vi "4461 - AI Read Data.vi"(8 "error in (no error)":errorcluster, 9 "sampling info":cluster{"Fs":dbl, "#s":dbl}={"Fs"=1000.0, "#s"=1000.0} {"Fs" format="%.2p"}, 10 "AI Block Size":i32=5000, 11 "AI task":refnum<k21>[](array[refnum])=["", ""]) -> (0 "error out":errorcluster, 1 "Backlog":u8(slide) scale=0.0..100.0, 2 "Input Signals":dbl[][](array[numeric]), 3 "Input Signals":waveform(dbl)[](array[waveform]))   [LabVIEW 2013]
uses:
  <vilib>/DAQmx/read.llb/DAQmx Read (Analog 1D Wfm NChan NSamp).vi
  <vilib>/DAQmx/miscellaneous.llb/DAQmx Fill In Error Info.vi
  <resource>/objmgr/daqmx.rc
panel:
  out "AvailSampPerChan 8":u32
  out "AvailSampPerChan 7":u32
  out "AvailSampPerChan 6":u32
  out "AvailSampPerChan 5":u32
  out "AvailSampPerChan 4":u32
  out "AvailSampPerChan 3":u32
  out "AvailSampPerChan 2":u32
  out "AvailSampPerChan":u32
  in  "AI Rate":dbl=10000.0 format="%.2f"
  in  "AI Buffer Size (s)":i32=10
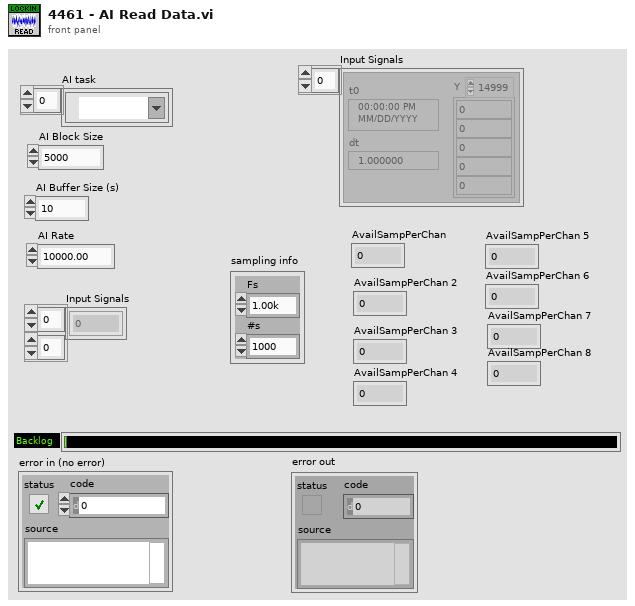
[diagram p1: front panel]
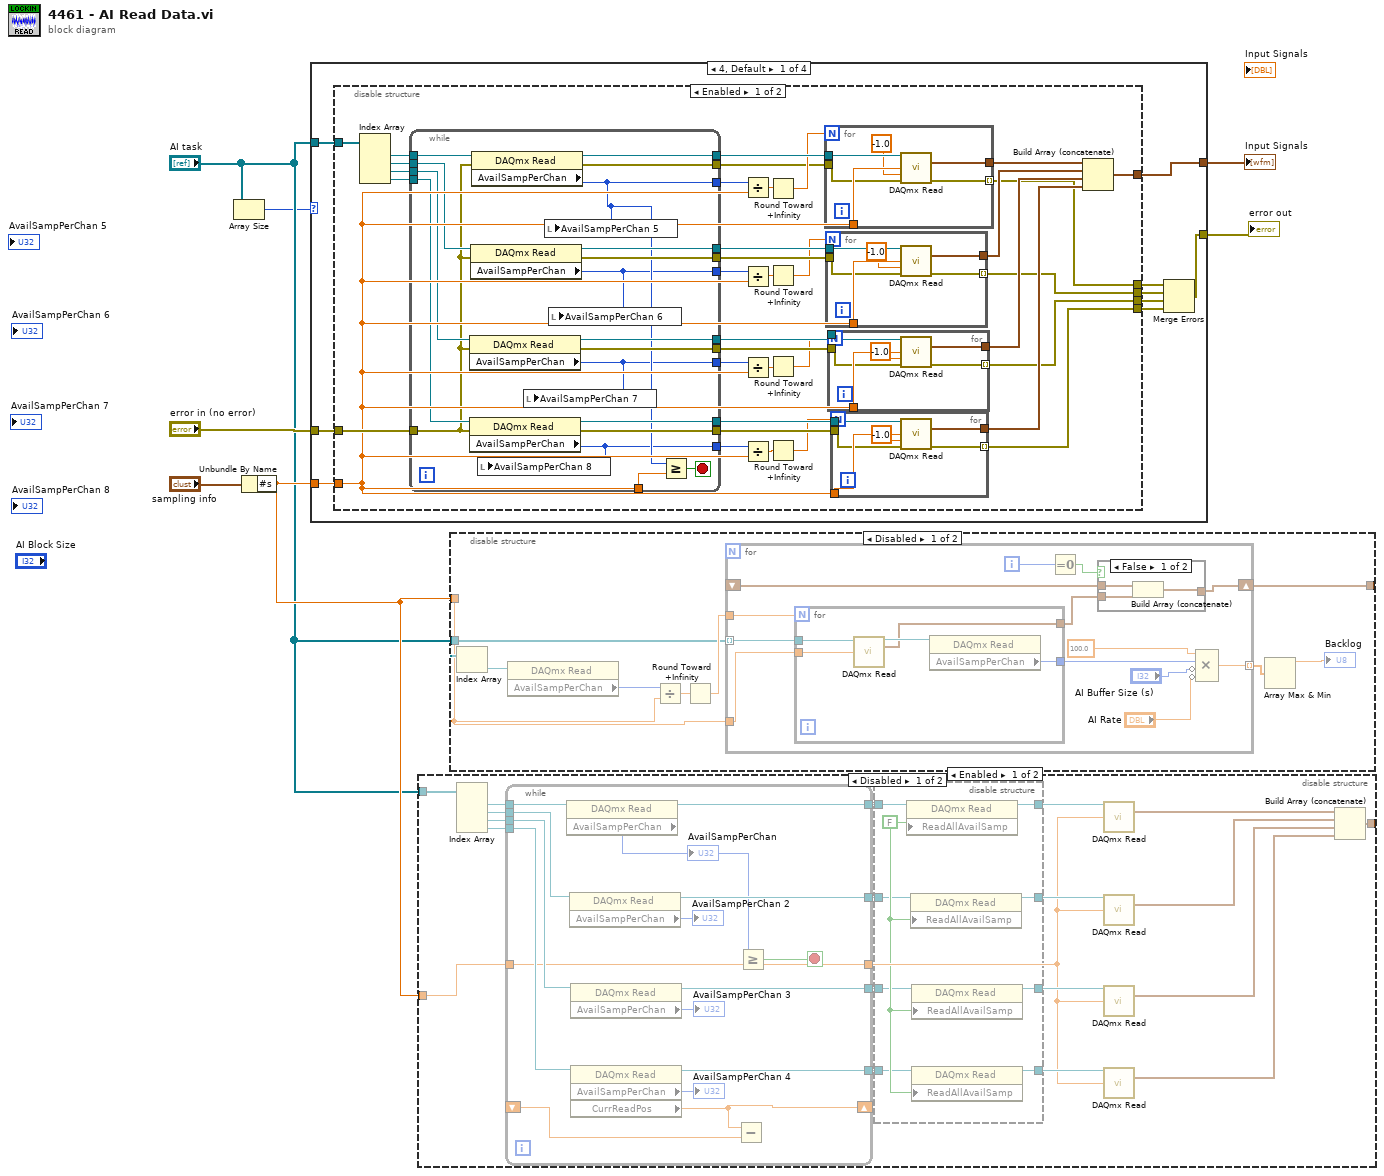
[diagram p0: block diagram]
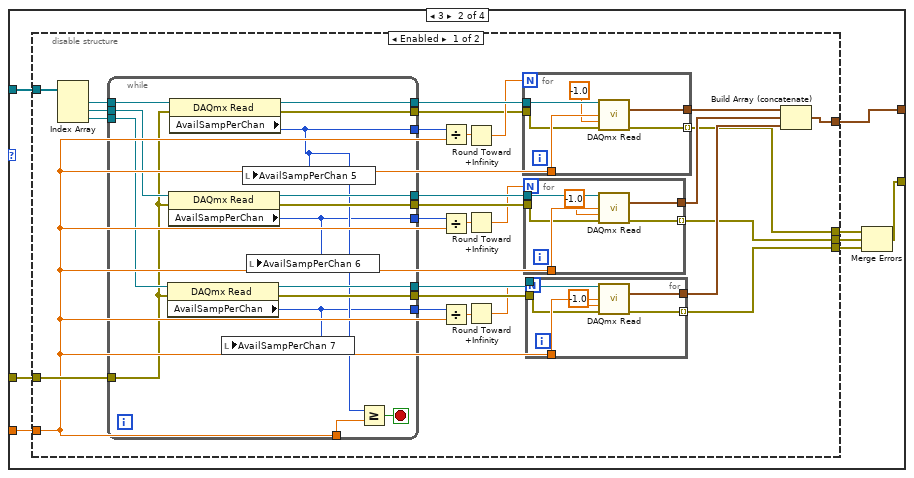
[diagram p3: hidden frame]
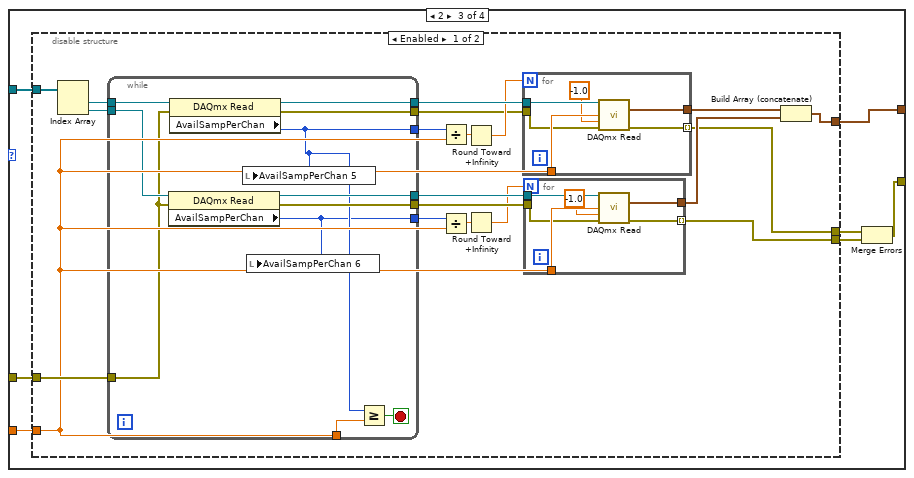
[diagram p5: hidden frame]
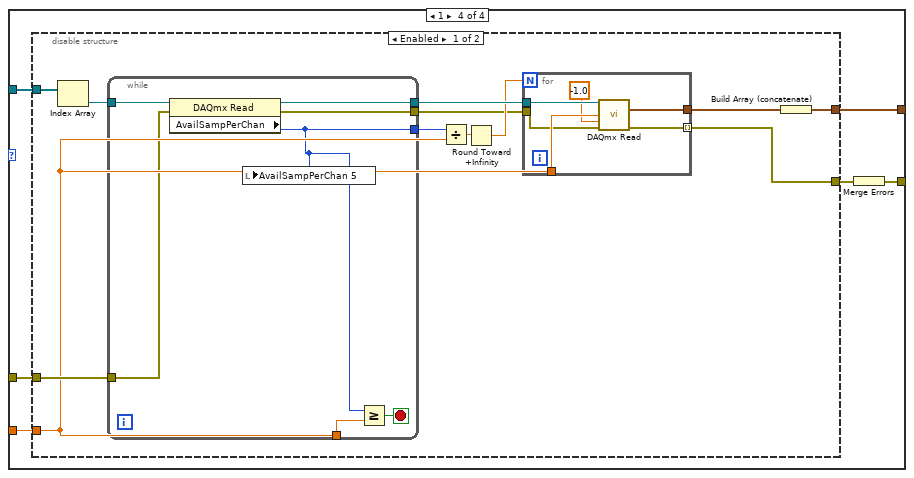
[diagram p7: hidden frame]
diagram:
  n1 = Array Size(array="AI task") -> (size(s)=w1:i32)
  n2 = Unbundle By Name("sampling info") -> ("#s"=w3:dbl)
  n3 = case shown="4, Default" w1 {
    tunnel: "AI task" -> [w16 w103 w171 w220]
    tunnel: [w15 w102 w170 w219] -> w6
    tunnel: "error in (no error)" -> [w14 w101 w169 w218]
    tunnel: [w12 w99 w167 w216] -> w4
    tunnel: w3 -> [w8 w96 w165 w215]
    frame 4, Default {
      n4 = disable-structure shown="Enabled" {
        disable-tunnel: w16 -> [w52 _]
        disable-tunnel: w8 -> [w17 _]
        disable-tunnel: [w31 _] -> w15
        disable-tunnel: w14 -> [w29 _]
        disable-tunnel: [w24 _] -> w13
        disable-tunnel: [w23 _] -> w11
        disable-tunnel: [w22 _] -> w10
        disable-tunnel: [w21 _] -> w9
        frame Enabled {
          n5 = Index Array(array=w52) -> (element #1=w44:refnum<k21>, element #2=w45:refnum<k21>, element #3=w46:refnum<k21>, element #4=w47:refnum<k21>)  [unwired: 4 in]
          n6 = while {
            tunnel: w47 -> [w71]
            tunnel: w46 -> [w70]
            tunnel: w45 -> [w69]
            tunnel: w44 -> [w68]
            tunnel: [w67] -> w43
            tunnel: [w66] -> w42
            tunnel: [w65] -> w41
            tunnel: [w64] -> w40
            tunnel: [w56] -> w39
            tunnel: [w53] -> w38
            tunnel: [w54] -> w37
            tunnel: [w55] -> w36
            tunnel: w29 -> [w57]
            tunnel: [w63] -> w28
            tunnel: [w62] -> w27
            tunnel: [w61] -> w26
            tunnel: [w60] -> w25
            tunnel: w17 -> [w59]
            stop <- w58 stop-if-true
            n7 = property class="DAQmx Read"(reference=w70, error in=w57) -> (reference out=w65:refnum<k21>, error out=w61:errorcluster, "AvailSampPerChan"=w54:u32)
            n8 = property class="DAQmx Read"(reference=w71, error in=w57) -> (reference out=w64:refnum<k21>, error out=w60:errorcluster, "AvailSampPerChan"=w53:u32)
            n9 = property class="DAQmx Read"(reference=w69, error in=w57) -> (reference out=w66:refnum<k21>, error out=w62:errorcluster, "AvailSampPerChan"=w55:u32)
            n10 = property class="DAQmx Read"(reference=w68, error in=w57) -> (reference out=w67:refnum<k21>, error out=w63:errorcluster, "AvailSampPerChan"=w56:u32)
            n11 = local write "AvailSampPerChan 8"(w53) -> ()
            n12 = local write "AvailSampPerChan 7"(w54) -> ()
            n13 = local write "AvailSampPerChan 5"(w56) -> ()
            n14 = local write "AvailSampPerChan 6"(w55) -> ()
            n15 = Greater Or Equal?(x=w56, y=w59) -> (x >= y?=w58:bool)
          }
          n16 = Divide(x=w39, y=w17) -> (x/y=w35:dbl)
          n17 = Divide(x=w36, y=w17) -> (x/y=w34:dbl)
          n18 = Divide(x=w37, y=w17) -> (x/y=w33:dbl)
          n19 = Divide(x=w38, y=w17) -> (x/y=w32:dbl)
          n20 = Round Toward +Infinity(x=w35) -> (ceil(x): smallest int >= x=w30:dbl)
          n21 = Round Toward +Infinity(x=w34) -> (ceil(x): smallest int >= x=w18:dbl)
          n22 = Round Toward +Infinity(x=w33) -> (ceil(x): smallest int >= x=w19:dbl)
          n23 = Round Toward +Infinity(x=w32) -> (ceil(x): smallest int >= x=w20:dbl)
          n24 = for {
            N: w30 -> [_]
            tunnel: [w95] -> w48
            tunnel: w43 -> [w94]
            tunnel: w17 -> [w93]
            tunnel: w28 -> [w92]
            tunnel: [w91] -> w24 mode=indexing
            n25 = call-poly <vilib>:"DAQmx Read.vi"("task/channels in"=w94, "number of samples per channel"=w93, "timeout"=-1.0, "error in"=w92) -> ("data"=w95:waveform(dbl)[], "error out"=w91:errorcluster)  [unwired: 9 in, 1 out]
          }
          n26 = for {
            N: w18 -> [_]
            tunnel: [w89] -> w49
            tunnel: w42 -> [w88]
            tunnel: w17 -> [w87]
            tunnel: w27 -> [w86]
            tunnel: [w85] -> w23 mode=indexing
            n27 = call-poly <vilib>:"DAQmx Read.vi"("task/channels in"=w88, "number of samples per channel"=w87, "timeout"=-1.0, "error in"=w86) -> ("data"=w89:waveform(dbl)[], "error out"=w85:errorcluster)  [unwired: 9 in, 1 out]
          }
          n28 = for {
            N: w19 -> [_]
            tunnel: [w83] -> w50
            tunnel: w41 -> [w82]
            tunnel: w17 -> [w81]
            tunnel: w26 -> [w80]
            tunnel: [w79] -> w22 mode=indexing
            n29 = call-poly <vilib>:"DAQmx Read.vi"("task/channels in"=w82, "number of samples per channel"=w81, "timeout"=-1.0, "error in"=w80) -> ("data"=w83:waveform(dbl)[], "error out"=w79:errorcluster)  [unwired: 9 in, 1 out]
          }
          n30 = for {
            N: w20 -> [_]
            tunnel: [w77] -> w51
            tunnel: w40 -> [w76]
            tunnel: w17 -> [w75]
            tunnel: w25 -> [w74]
            tunnel: [w73] -> w21 mode=indexing
            n31 = call-poly <vilib>:"DAQmx Read.vi"("task/channels in"=w76, "number of samples per channel"=w75, "timeout"=-1.0, "error in"=w74) -> ("data"=w77:waveform(dbl)[], "error out"=w73:errorcluster)  [unwired: 9 in, 1 out]
          }
          n32 = Build Array (concatenate)(w48, w49, w50, w51) -> (w31:waveform(dbl)[])
        }
        frame Disabled {
        }
      }
      n33 = Merge Errors(w13, w11, w10, w9) -> (w12:errorcluster)
    }
    frame 3 {
      n34 = disable-structure shown="Enabled" {
        disable-tunnel: w103 -> [w131 _]
        disable-tunnel: w96 -> [w104 _]
        disable-tunnel: [w115 _] -> w102
        disable-tunnel: w101 -> [w113 _]
        disable-tunnel: [w109 _] -> w100
        disable-tunnel: [w108 _] -> w98
        disable-tunnel: [w107 _] -> w97
        frame Enabled {
          n35 = Index Array(array=w131) -> (element #1=w125:refnum<k21>, element #2=w126:refnum<k21>, element #3=w127:refnum<k21>)  [unwired: 3 in]
          n36 = while {
            tunnel: w127 -> [w146]
            tunnel: w126 -> [w145]
            tunnel: w125 -> [w144]
            tunnel: [w143] -> w124
            tunnel: [w142] -> w123
            tunnel: [w141] -> w122
            tunnel: [w134] -> w121
            tunnel: [w132] -> w120
            tunnel: [w133] -> w119
            tunnel: w113 -> [w135]
            tunnel: [w140] -> w112
            tunnel: [w139] -> w111
            tunnel: [w138] -> w110
            tunnel: w104 -> [w137]
            stop <- w136 stop-if-true
            n37 = property class="DAQmx Read"(reference=w146, error in=w135) -> (reference out=w141:refnum<k21>, error out=w138:errorcluster, "AvailSampPerChan"=w132:u32)
            n38 = property class="DAQmx Read"(reference=w145, error in=w135) -> (reference out=w142:refnum<k21>, error out=w139:errorcluster, "AvailSampPerChan"=w133:u32)
            n39 = property class="DAQmx Read"(reference=w144, error in=w135) -> (reference out=w143:refnum<k21>, error out=w140:errorcluster, "AvailSampPerChan"=w134:u32)
            n40 = local write "AvailSampPerChan 7"(w132) -> ()
            n41 = local write "AvailSampPerChan 5"(w134) -> ()
            n42 = local write "AvailSampPerChan 6"(w133) -> ()
            n43 = Greater Or Equal?(x=w134, y=w137) -> (x >= y?=w136:bool)
          }
          n44 = Divide(x=w121, y=w104) -> (x/y=w118:dbl)
          n45 = Divide(x=w119, y=w104) -> (x/y=w117:dbl)
          n46 = Divide(x=w120, y=w104) -> (x/y=w116:dbl)
          n47 = Round Toward +Infinity(x=w118) -> (ceil(x): smallest int >= x=w114:dbl)
          n48 = Round Toward +Infinity(x=w117) -> (ceil(x): smallest int >= x=w105:dbl)
          n49 = Round Toward +Infinity(x=w116) -> (ceil(x): smallest int >= x=w106:dbl)
          n50 = for {
            N: w114 -> [_]
            tunnel: [w164] -> w128
            tunnel: w124 -> [w163]
            tunnel: w104 -> [w162]
            tunnel: w112 -> [w161]
            tunnel: [w160] -> w109 mode=indexing
            n51 = call-poly <vilib>:"DAQmx Read.vi"("task/channels in"=w163, "number of samples per channel"=w162, "timeout"=-1.0, "error in"=w161) -> ("data"=w164:waveform(dbl)[], "error out"=w160:errorcluster)  [unwired: 9 in, 1 out]
          }
          n52 = for {
            N: w105 -> [_]
            tunnel: [w158] -> w129
            tunnel: w123 -> [w157]
            tunnel: w104 -> [w156]
            tunnel: w111 -> [w155]
            tunnel: [w154] -> w108 mode=indexing
            n53 = call-poly <vilib>:"DAQmx Read.vi"("task/channels in"=w157, "number of samples per channel"=w156, "timeout"=-1.0, "error in"=w155) -> ("data"=w158:waveform(dbl)[], "error out"=w154:errorcluster)  [unwired: 9 in, 1 out]
          }
          n54 = for {
            N: w106 -> [_]
            tunnel: [w152] -> w130
            tunnel: w122 -> [w151]
            tunnel: w104 -> [w150]
            tunnel: w110 -> [w149]
            tunnel: [w148] -> w107 mode=indexing
            n55 = call-poly <vilib>:"DAQmx Read.vi"("task/channels in"=w151, "number of samples per channel"=w150, "timeout"=-1.0, "error in"=w149) -> ("data"=w152:waveform(dbl)[], "error out"=w148:errorcluster)  [unwired: 9 in, 1 out]
          }
          n56 = Build Array (concatenate)(w128, w129, w130) -> (w115:waveform(dbl)[])
        }
        frame Disabled {
        }
      }
      n57 = Merge Errors(w100, w98, w97) -> (w99:errorcluster)
    }
    frame 2 {
      n58 = disable-structure shown="Enabled" {
        disable-tunnel: w171 -> [w191 _]
        disable-tunnel: w165 -> [w172 _]
        disable-tunnel: [w180 _] -> w170
        disable-tunnel: w169 -> [w178 _]
        disable-tunnel: [w175 _] -> w168
        disable-tunnel: [w174 _] -> w166
        frame Enabled {
          n59 = Index Array(array=w191) -> (element #1=w187:refnum<k21>, element #2=w188:refnum<k21>)  [unwired: 2 in]
          n60 = while {
            tunnel: w188 -> [w202]
            tunnel: w187 -> [w201]
            tunnel: [w200] -> w186
            tunnel: [w199] -> w185
            tunnel: [w193] -> w184
            tunnel: [w192] -> w183
            tunnel: w178 -> [w194]
            tunnel: [w198] -> w177
            tunnel: [w197] -> w176
            tunnel: w172 -> [w196]
            stop <- w195 stop-if-true
            n61 = property class="DAQmx Read"(reference=w202, error in=w194) -> (reference out=w199:refnum<k21>, error out=w197:errorcluster, "AvailSampPerChan"=w192:u32)
            n62 = property class="DAQmx Read"(reference=w201, error in=w194) -> (reference out=w200:refnum<k21>, error out=w198:errorcluster, "AvailSampPerChan"=w193:u32)
            n63 = local write "AvailSampPerChan 5"(w193) -> ()
            n64 = local write "AvailSampPerChan 6"(w192) -> ()
            n65 = Greater Or Equal?(x=w193, y=w196) -> (x >= y?=w195:bool)
          }
          n66 = Divide(x=w184, y=w172) -> (x/y=w182:dbl)
          n67 = Divide(x=w183, y=w172) -> (x/y=w181:dbl)
          n68 = Round Toward +Infinity(x=w182) -> (ceil(x): smallest int >= x=w179:dbl)
          n69 = Round Toward +Infinity(x=w181) -> (ceil(x): smallest int >= x=w173:dbl)
          n70 = for {
            N: w179 -> [_]
            tunnel: [w214] -> w189
            tunnel: w186 -> [w213]
            tunnel: w172 -> [w212]
            tunnel: w177 -> [w211]
            tunnel: [w210] -> w175 mode=indexing
            n71 = call-poly <vilib>:"DAQmx Read.vi"("task/channels in"=w213, "number of samples per channel"=w212, "timeout"=-1.0, "error in"=w211) -> ("data"=w214:waveform(dbl)[], "error out"=w210:errorcluster)  [unwired: 9 in, 1 out]
          }
          n72 = for {
            N: w173 -> [_]
            tunnel: [w208] -> w190
            tunnel: w185 -> [w207]
            tunnel: w172 -> [w206]
            tunnel: w176 -> [w205]
            tunnel: [w204] -> w174 mode=indexing
            n73 = call-poly <vilib>:"DAQmx Read.vi"("task/channels in"=w207, "number of samples per channel"=w206, "timeout"=-1.0, "error in"=w205) -> ("data"=w208:waveform(dbl)[], "error out"=w204:errorcluster)  [unwired: 9 in, 1 out]
          }
          n74 = Build Array (concatenate)(w189, w190) -> (w180:waveform(dbl)[])
        }
        frame Disabled {
        }
      }
      n75 = Merge Errors(w168, w166) -> (w167:errorcluster)
    }
    frame 1 {
      n76 = disable-structure shown="Enabled" {
        disable-tunnel: w220 -> [w232 _]
        disable-tunnel: w215 -> [w221 _]
        disable-tunnel: [w226 _] -> w219
        disable-tunnel: w218 -> [w224 _]
        disable-tunnel: [w222 _] -> w217
        frame Enabled {
          n77 = Index Array(array=w232) -> (element=w230:refnum<k21>)  [unwired: 1 in]
          n78 = while {
            tunnel: w230 -> [w239]
            tunnel: [w238] -> w229
            tunnel: [w233] -> w228
            tunnel: w224 -> [w234]
            tunnel: [w237] -> w223
            tunnel: w221 -> [w236]
            stop <- w235 stop-if-true
            n79 = property class="DAQmx Read"(reference=w239, error in=w234) -> (reference out=w238:refnum<k21>, error out=w237:errorcluster, "AvailSampPerChan"=w233:u32)
            n80 = local write "AvailSampPerChan 5"(w233) -> ()
            n81 = Greater Or Equal?(x=w233, y=w236) -> (x >= y?=w235:bool)
          }
          n82 = Divide(x=w228, y=w221) -> (x/y=w227:dbl)
          n83 = Round Toward +Infinity(x=w227) -> (ceil(x): smallest int >= x=w225:dbl)
          n84 = for {
            N: w225 -> [_]
            tunnel: [w245] -> w231
            tunnel: w229 -> [w244]
            tunnel: w221 -> [w243]
            tunnel: w223 -> [w242]
            tunnel: [w241] -> w222 mode=indexing
            n85 = call-poly <vilib>:"DAQmx Read.vi"("task/channels in"=w244, "number of samples per channel"=w243, "timeout"=-1.0, "error in"=w242) -> ("data"=w245:waveform(dbl)[], "error out"=w241:errorcluster)  [unwired: 9 in, 1 out]
          }
          n86 = Build Array (concatenate)(w231) -> (w226:waveform(dbl)[])
        }
        frame Disabled {
        }
      }
      n87 = Merge Errors(w217) -> (w216:errorcluster)
    }
  }
  "Input Signals" <- w6
  "error out" <- w4
  n88 = disable-structure shown="Disabled" {
    disable-tunnel: "AI task" -> [w265 _]
    disable-tunnel: w3 -> [w247 _]
    disable-tunnel: [w256 _] -> _
    frame Disabled {
      n89 = Index Array(array=w265) -> (element #1=w255:refnum<k21>, element #2=w250:refnum<k21>, element #3=w249:refnum<k21>, element #4=w248:refnum<k21>)  [unwired: 4 in]
      n90 = while {
        tunnel: w255 -> [w282]
        tunnel: [w281] -> w254
        tunnel: [w280] -> w253
        tunnel: [w279] -> w252
        tunnel: [w278] -> w251
        tunnel: w250 -> [w277]
        tunnel: w249 -> [w276]
        tunnel: w248 -> [w275]
        tunnel: w247 -> [w266]
        shift-right: [w269] -> _
        shift-left: _ -> [w268]
        tunnel: [w266] -> w246
        stop <- w270 stop-if-true
        n91 = property class="DAQmx Read"(reference=w282) -> (reference out=w281:refnum<k21>, "AvailSampPerChan"=w271:u32)  [unwired: 1 in, 1 out]
        "AvailSampPerChan" <- w271
        n92 = property class="DAQmx Read"(reference=w277) -> (reference out=w280:refnum<k21>, "AvailSampPerChan"=→"AvailSampPerChan 2":u32)  [unwired: 1 in, 1 out]
        n93 = property class="DAQmx Read"(reference=w276) -> (reference out=w279:refnum<k21>, "AvailSampPerChan"=→"AvailSampPerChan 3":u32)  [unwired: 1 in, 1 out]
        n94 = property class="DAQmx Read"(reference=w275) -> (reference out=w278:refnum<k21>, "AvailSampPerChan"=→"AvailSampPerChan 4":u32, "CurrReadPos"=w269:dbl)  [unwired: 1 in, 1 out]
        n95 = Subtract(x=w269, y=w268) -> (x-y=w267:dbl)
        n96 = Greater Or Equal?(x=w271, y=w266) -> (x >= y?=w270:bool)
      }
      n97 = disable-structure shown="Enabled" {
        disable-tunnel: w254 -> [w291 w295]
        disable-tunnel: [w290 w295] -> w264
        disable-tunnel: [w289 w292] -> w263
        disable-tunnel: [w288 w293] -> w262
        disable-tunnel: [w287 w294] -> w261
        disable-tunnel: w253 -> [w285 w294]
        disable-tunnel: w252 -> [w284 w293]
        disable-tunnel: w251 -> [w283 w292]
        frame Enabled {
          w286 = FALSE ("ReadAllAvailSamp")
          n98 = property class="DAQmx Read"(reference=w291, "ReadAllAvailSamp"=w286) -> (reference out=w290:refnum<k21>)  [unwired: 1 in, 1 out]
          n99 = property class="DAQmx Read"(reference=w285, "ReadAllAvailSamp"=w286) -> (reference out=w287:refnum<k21>)  [unwired: 1 in, 1 out]
          n100 = property class="DAQmx Read"(reference=w284, "ReadAllAvailSamp"=w286) -> (reference out=w288:refnum<k21>)  [unwired: 1 in, 1 out]
          n101 = property class="DAQmx Read"(reference=w283, "ReadAllAvailSamp"=w286) -> (reference out=w289:refnum<k21>)  [unwired: 1 in, 1 out]
        }
        frame Disabled {
        }
      }
      n102 = call-poly <vilib>:"DAQmx Read.vi"("task/channels in"=w264, "number of samples per channel"=w246) -> ("data"=w260:waveform(dbl)[])  [unwired: 11 in, 2 out]
      n103 = call-poly <vilib>:"DAQmx Read.vi"("task/channels in"=w261, "number of samples per channel"=w246) -> ("data"=w259:waveform(dbl)[])  [unwired: 11 in, 2 out]
      n104 = call-poly <vilib>:"DAQmx Read.vi"("task/channels in"=w262, "number of samples per channel"=w246) -> ("data"=w258:waveform(dbl)[])  [unwired: 11 in, 2 out]
      n105 = call-poly <vilib>:"DAQmx Read.vi"("task/channels in"=w263, "number of samples per channel"=w246) -> ("data"=w257:waveform(dbl)[])  [unwired: 11 in, 2 out]
      n106 = Build Array (concatenate)(w260, w259, w258, w257) -> (w256:waveform(dbl)[])
    }
    frame Enabled {
    }
  }
  n107 = disable-structure shown="Disabled" {
    disable-tunnel: [w298 _] -> _
    disable-tunnel: "AI task" -> [w297 _]
    disable-tunnel: w3 -> [w296 _]
    frame Disabled {
      n108 = Index Array(array=w297) -> (element=w302:refnum<k21>)  [unwired: 1 in]
      n109 = property class="DAQmx Read"(reference=w302) -> ("AvailSampPerChan"=w301:u32)  [unwired: 1 in, 2 out]
      n110 = Divide(x=w301, y=w296) -> (x/y=w300:dbl)
      n111 = Round Toward +Infinity(x=w300) -> (ceil(x): smallest int >= x=w299:dbl)
      n112 = for {
        tunnel: w297 -> [w309] mode=indexing
        tunnel: [w315] -> w304 mode=indexing
        shift-right: [w310] -> w298
        shift-left: _ -> [w312]
        tunnel: w299 -> [w308]
        tunnel: w296 -> [w307]
        i -> [w313]
        n113 = for {
          N: w308 -> [_]
          tunnel: [w325] -> w311
          tunnel: [w324] -> w317
          tunnel: w309 -> [w323]
          tunnel: w307 -> [w322]
          n114 = call-poly <vilib>:"DAQmx Read.vi"("task/channels in"=w323, "number of samples per channel"=w322) -> ("task out"=w326:refnum<k21>, "data"=w325:waveform(dbl)[])  [unwired: 11 in, 1 out]
          n115 = property class="DAQmx Read"(reference=w326) -> ("AvailSampPerChan"=w324:u32)  [unwired: 1 in, 2 out]
        }
        n116 = Equal To 0?(x=w313) -> (x = 0?=w314:bool)
        n117 = case shown="False" w314 {
          tunnel: w312 -> [w318 _]
          tunnel: w311 -> [w320 w321]
          tunnel: [w319 w321] -> w310
          frame False {
            n118 = Build Array (concatenate)(w318, w320) -> (w319:waveform(dbl)[])
          }
          frame True {
          }
        }
        n119 = Compound Arithmetic op=MULTIPLY(100.0 ("value"), w317, invert "AI Buffer Size (s)", invert "AI Rate") -> (w315:dbl)
      }
      n120 = Array Max & Min(array=w304) -> (max value=→"Backlog":dbl)  [unwired: 3 out]
    }
    frame Enabled {
    }
  }
